vi "Get State from Routing Channel.vi"(8 "error in (no error)":errorcluster, 10 "State":string, 11 "Channel Ref in":T3 format="%.0x") -> (0 "error out":errorcluster, 2 "Routing State":T1, 3 "Channel Ref out":T3=18446744073709551615 format="%.0x")   [LabVIEW 2017, in "Switch Scripting.lvlib"]
uses:
  Switch Scripting.lvlib
  <vilib>/NI Veristand/Custom Device API/Custom Device Item Ref.ctl
  Routing State.ctl
  Connection.ctl
  NationalInstruments.VeriStand.SystemDefinitionAPI
  Shared/Constants.vi
  Shared/Switch Shared.lvlib
  <vilib>/NI VeriStand/Custom Device API/Custom Device API.lvlib
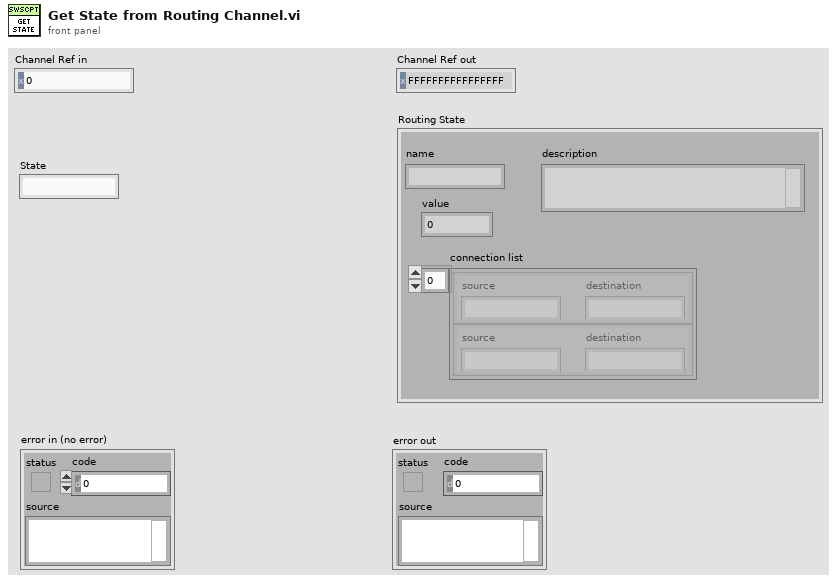
[diagram p1: front panel]
types:
  T1 = typedef "Switch Scripting.lvlib/Routing State.ctl" = cluster{"name":string, "description":string, "value":i32, "connection list":T2[]}
  T2 = typedef "Switch Scripting.lvlib/Connection.ctl" = cluster{"source":string, "destination":string}
  T3 = typedef "Custom Device API.lvlib/Custom Device Item Ref.ctl" = u64
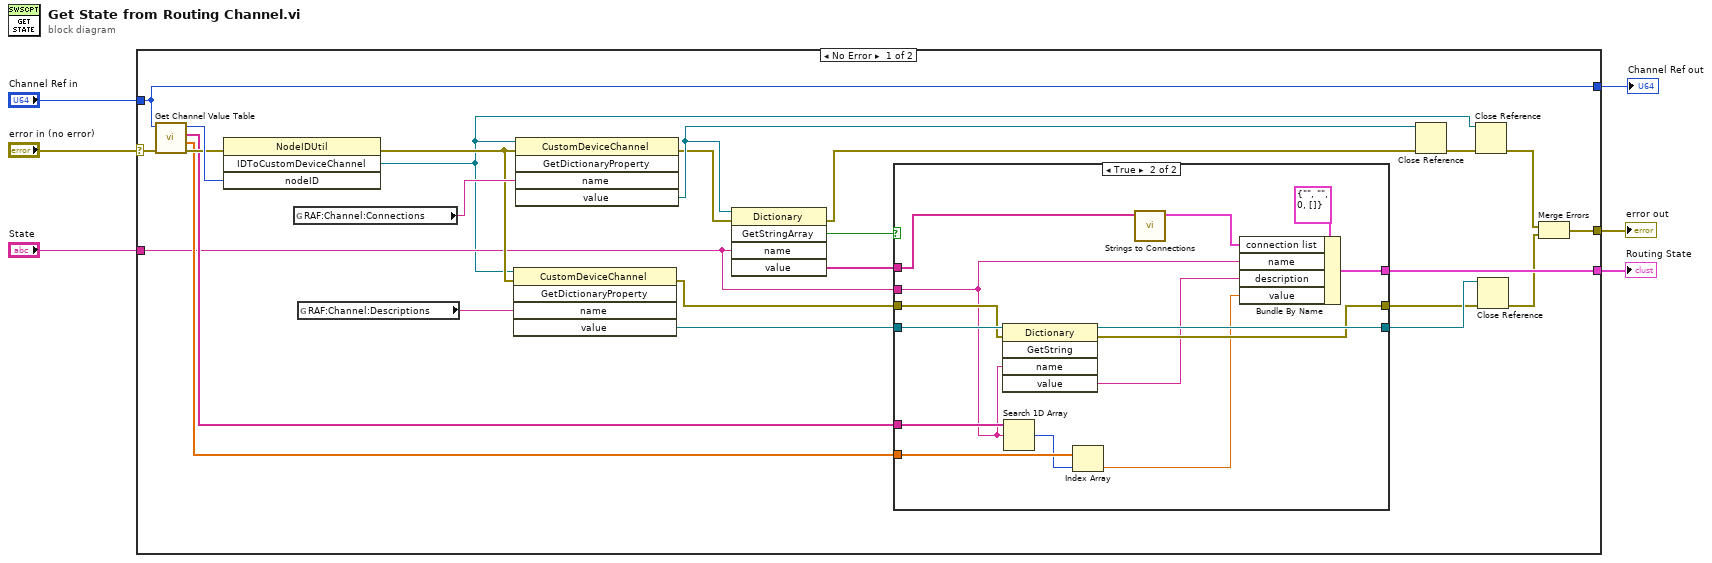
[diagram p0: block diagram]
diagram:
  n1 = case shown="No Error" "error in (no error)" {
    selector: "error in (no error)" -> [w28 w49]
    tunnel: [w14 w49] -> w2
    tunnel: "Channel Ref in" -> [w30 w48]
    tunnel: [w30 w48] -> w1
    tunnel: [w31 _] -> w3
    tunnel: "State" -> [w9 _]
    frame No Error {
      n2 = call "Get Channel Value Table.vi"("error in (no error)"=w28, "Channel Ref in"=w30) -> ("error out"=w27:errorcluster, "Values"=w25:dbl[], "States"=w26:string[], "Channel Ref out"=w29:T3)  [unwired: 6 in]
      n3 = invoke class="NodeIDUtil" method="IDToCustomDeviceChannel"(error in=w27, "nodeID"=w29) -> (error out=w20:errorcluster, "IDToCustomDeviceChannel"=w7:refnum<k24>)  [unwired: 2 in, 2 out]
      n4 = global read "Constants.vi" "RAF:Channel:Connections"() -> (w24:string)
      n5 = global read "Constants.vi" "RAF:Channel:Descriptions"() -> (w23:string)
      n6 = invoke class="CustomDeviceChannel" method="GetDictionaryProperty"(reference=w7, error in=w20, "name"=w23) -> (error out=w19:errorcluster, "value"=w22:refnum<k24>)  [unwired: 2 in, 3 out]
      n7 = invoke class="CustomDeviceChannel" method="GetDictionaryProperty"(reference=w7, error in=w20, "name"=w24) -> (error out=w12:errorcluster, "value"=w13:refnum<k24>)  [unwired: 2 in, 3 out]
      n8 = invoke class="Dictionary" method="GetStringArray"(reference=w13, error in=w12, "name"=w9) -> (error out=w10:errorcluster, "GetStringArray"=w8:bool, "value"=w11:string[])  [unwired: 2 in, 2 out]
      n9 = case shown="True" w8 {
        tunnel: [_ w47] -> w31
        tunnel: w26 -> [_ w46]
        tunnel: w25 -> [_ w45]
        tunnel: w22 -> [w33 w44]
        tunnel: [w33 w43] -> w21
        tunnel: w19 -> [w32 w42]
        tunnel: [w32 w41] -> w18
        tunnel: w11 -> [_ w40]
        tunnel: w9 -> [_ w34]
        frame False {
        }
        frame True {
          n10 = invoke class="Dictionary" method="GetString"(reference=w44, error in=w42, "name"=w34) -> (reference out=w43:refnum<k24>, error out=w41:errorcluster, "value"=w36:string)  [unwired: 2 in, 2 out]
          n11 = Search 1D Array(1D array=w46, element=w34) -> (index of element=w38:i32)  [unwired: 1 in]
          n12 = Index Array(array=w45, index=w38) -> (element=w37:dbl)
          n13 = call "Strings to Connections.vi"("connection strings"=w40) -> ("connection list"=w35:T2[])  [unwired: 10 in]
          n14 = Bundle By Name(cluster=T1 {"name"="", "description"="", "value"=0, "connection list"=[]} ("Routing State"), "connection list"=w35, "name"=w34, "description"=w36, "value"=w37) -> (w47:T1)
        }
      }
      n15 = Close Reference(reference=w13, error in (no error)=w10) -> (error out=w17:errorcluster)
      n16 = Close Reference(reference=w7, error in (no error)=w17) -> (error out=w16:errorcluster)
      n17 = Close Reference(reference=w21, error in (no error)=w18) -> (error out=w15:errorcluster)
      n18 = Merge Errors(w16, w15) -> (w14:errorcluster)
    }
    frame Error {
    }
  }
  "Channel Ref out" <- w1
  "error out" <- w2
  "Routing State" <- w3
